vi "parse TDMS file.vi"(8 "error in":errorcluster, 9 "channel name(s) in":string[](array[string]), 10 "group names in":string[](array[string]), 11 "file path":path) -> (0 "error out":errorcluster, 1 "channel names":string[](array[string]), 2 "group names":string[](array[string]), 3 "Array":dbl[][](array[numeric]), 5 "property values":string[](array[string]), 7 "property names":string[](array[string]))   [LabVIEW 2015, in "tdms logger tests.lvlib"]
uses:
  tdms logger tests.lvlib
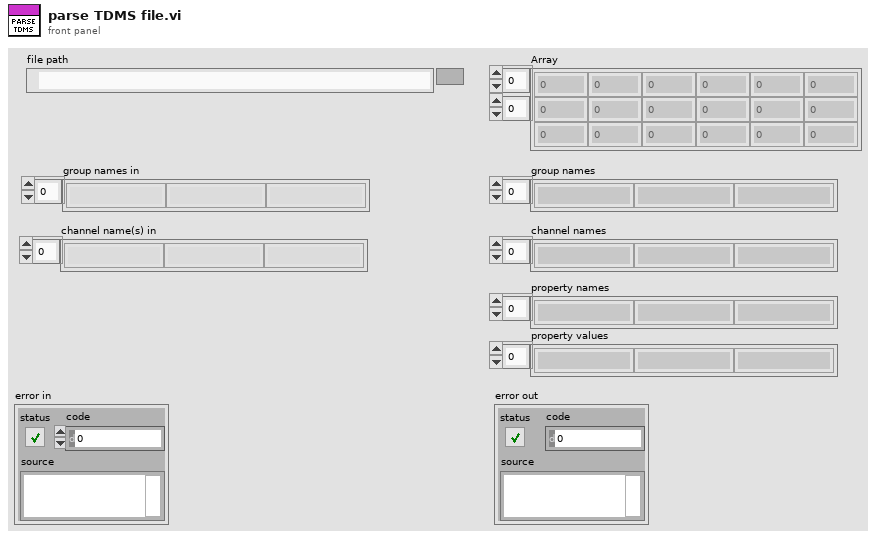
[diagram p1: front panel]
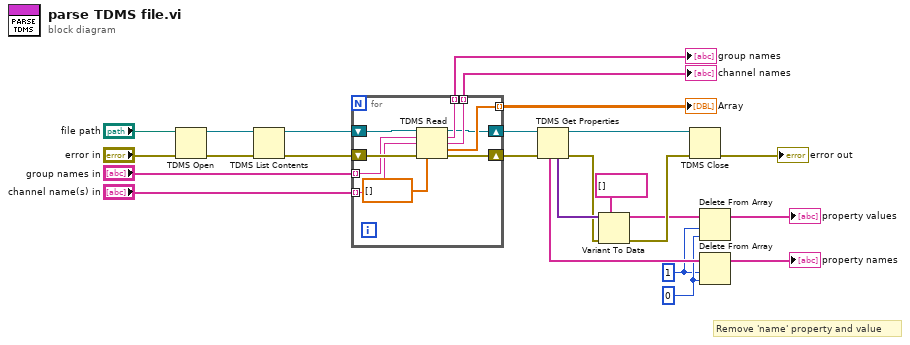
[diagram p0: block diagram]
diagram:
  w2 = 0 ("length")
  w1 = 1 ("length")
  # "Remove 'name' property and value"
  n1 = TDMS Open(8:"error in", 11:"file path") -> (0:w23:errorcluster, 3:w24:refnum<k34>)  [unwired: 5 in]
  n2 = TDMS List Contents(4:w23, 7:w24) -> (0:w21:errorcluster, 3:w22:refnum<k34>)  [unwired: 1 in, 2 out]
  n3 = for {
    tunnel: "group names in" -> [w33] mode=indexing
    tunnel: "channel name(s) in" -> [w32] mode=indexing
    tunnel: [w30] -> w18 mode=indexing
    shift-right: [w29] -> w11
    shift-left: w21 -> [w34]
    tunnel: [w28] -> w16 mode=indexing
    tunnel: [w27] -> w15 mode=indexing
    shift-right: [w26] -> w13
    shift-left: w22 -> [w35]
    n4 = TDMS Read(0:w35, 5:w33, 7:w32, 11:w34, 12:dbl[] []) -> (4:w26:refnum<k34>, 6:w28:string, 8:w27:string, 10:w30:dbl[], 15:w29:errorcluster)  [unwired: 3 in, 1 out]
  }
  "group names" <- w16
  "Array" <- w18
  "channel names" <- w15
  n5 = TDMS Get Properties(8:w11, 11:w13) -> (0:w8:errorcluster, 3:w12:refnum<k34>, 4:w10:variant[], 6:w4:string[])  [unwired: 4 in, 2 out]
  n6 = Variant To Data(error in=w8, type=string[] [] ("property values"), Variant=w10) -> (data=w6:string[], error out=w7:errorcluster)
  n7 = TDMS Close(8:w7, 11:w12) -> (0:→"error out":errorcluster)  [unwired: 1 out]
  n8 = Delete From Array(array=w6, length=w1, index=w2) -> (array with subset deleted=→"property values":string[])  [unwired: 1 out]
  n9 = Delete From Array(array=w4, length=w1, index=w2) -> (array with subset deleted=→"property names":string[])  [unwired: 1 out]
